vi "SLSC_Example_AsyscRTEnginer.vi"(10 "Parameters":variant, 11 "Process":refnum<class "Process.lvclass">) -> ()   [LabVIEW 2020, in "SLSC EDS Engine.lvlib"]
uses:
  SLSC EDS Engine.lvlib
  <vilib>/NI/NIVS Inline Async API/_VS Inline Async API/Process/Process.lvclass
  Types/Async Engine State Control.ctl
  Shared/Compiled.Settings
  Shared/SLSC Static Settings.ctl
  SLSC CD API/SLSC CD Engine/SLSC Dynamic Channel.ctl
  SLSC CD API/SLSC CD Engine/SLSC Datatype.ctl
  <vilib>/NI/NIVS Inline Async API/_VS Inline Async API/Process/Process.lvclass/Process.ctl
  <vilib>/NI/NIVS Inline Async API/_Data Access Engine/Access Type Classes/Read/Read.lvclass/Read.ctl
  <vilib>/NI/NIVS Inline Async API/_Data Access Engine/Access Type Classes/ReadWrite/ReadWrite.lvclass/ReadWrite.ctl
  <vilib>/NI/NIVS Inline Async API/_Data Access Engine/Access Type Classes/Write/Write.lvclass/Write.ctl
  <vilib>/NI/NIVS Inline Async API/_Data Access Engine/Data Access Engine/Methods/Read.Data.Detect.vi
  <vilib>/NI/NIVS Inline Async API/_Data Access Engine/Data Access Engine/Methods/Write.Data.vi
  <vilib>/NI/NIVS Inline Async API/_Data Access Engine/Data Access Engine/Methods/ReadWrite.Data.vi
  <vilib>/NI/NIVS Inline Async API/_VS Inline Async API/Process/Data Member Access/Read Data Access.vi
  <vilib>/NI/NIVS Inline Async API/_VS Inline Async API/Error Handling Process/SubVIs/Error.ConvertArray.vi
  <vilib>/NI/NIVS Inline Async API/_Data Access Engine/Access Type Classes/Read/Read.ProcessData.Detect.vi
  <vilib>/NI/NIVS Inline Async API/_Data Access Engine/Access Type Classes/Write/Write.ProcessData.vi
  SLSC CD API/SLSC CD Shared/SLSC Define Resource Name.vi
  <vilib>/NI/NIVS Inline Async API/_Data Access Engine/Access Type Classes/ReadWrite/ReadWrite.ProcessData.vi
  <vilib>/NI/NIVS Inline Async API/_Data Access Engine/Access Type Classes/Write/Write.Buffer.vi
  <vilib>/NI/NIVS Inline Async API/_Data Access Engine/Access Type Classes/Write/Write.Commit.vi
  Shared/Constants.vi
  <vilib>/NI/NIVS Inline Async API/_Data Access Engine/Data Access Engine/Methods/Write.Lookup.vi
  <vilib>/NI/NIVS Inline Async API/_Data Access Engine/Data Access Engine/Methods/Read.Lookup.vi
  <vilib>/NI/NIVS Inline Async API/_Data Access Engine/Data Access Engine/Methods/ReadWrite.Lookup.vi
  <vilib>/SLSC/Initialize Session with Devices.vi
  <vilib>/SLSC/Set Generic Property.vi
  <vilib>/SLSC/Set Generic Property (Bool).vi
  <vilib>/SLSC/Set Generic Property (DBL).vi
  <vilib>/SLSC/Set Generic Property (I32).vi
  <vilib>/SLSC/Set Generic Property (I64).vi
  <vilib>/SLSC/Set Generic Property (String).vi
  <vilib>/SLSC/Set Generic Property (U32).vi
  <vilib>/SLSC/Set Generic Property (U64).vi
  SLSC CD API/SLSC CD Shared/SLSC Error Suppression.vi
  <vilib>/SLSC/Commit Properties.vi
  <vilib>/SLSC/Commit Properties for Devices.vi
  <vilib>/SLSC/Execute Command.vi
  <vilib>/SLSC/Execute Device Command.vi
  <vilib>/SLSC/Execute Phys Chan Command.vi
  <vilib>/SLSC/Get Generic Property.vi
  <vilib>/SLSC/Get Generic Property (Bool).vi
  <vilib>/SLSC/Get Generic Property (DBL).vi
  <vilib>/SLSC/Get Generic Property (I32).vi
  <vilib>/SLSC/Get Generic Property (I64).vi
  <vilib>/SLSC/Get Generic Property (String).vi
  <vilib>/SLSC/Get Generic Property (U32).vi
  <vilib>/SLSC/Get Generic Property (U64).vi
  <vilib>/SLSC/Close Session.vi
  <vilib>/NI/NIVS Inline Async API/_Data Access Engine/Data Access Engine/Data Access Engine.lvclass
  <vilib>/NI VeriStand/Custom Device Tools/Custom Device Utility Library/Custom Device Utility Library.lvlib
  <vilib>/SLSC/SLSC.lvlib
  Shared/SLSC EDS Shared.lvlib
  SLSC CD API/SLSC CD Shared/SLSC CD Shared.lvlib
  SLSC CD API/SLSC CD Engine/SLSC CD Engine.lvlib
  <vilib>/NI/NIVS Inline Async API/_Data Access Engine/Access Type Classes/Write/Write.lvclass
panel:
  out "LoopRate(ms)":u32=50
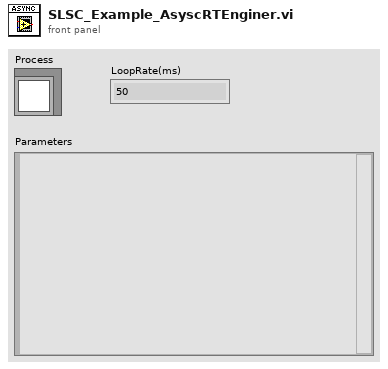
[diagram p1: front panel]
types:
  T1 = typedef "SLSC EDS Engine.lvlib/Async Engine State Control.ctl" = enum16{"Initialize", "Configure", "Run", "Reset", "Shutdown"}
  T2 = typedef "SLSC EDS Shared.lvlib/Compiled.Settings" = cluster{"Name":string, "SLSC Name or IP Address":string, "Slot #":i32, "Configuration Data":T3, "SLSC Get/Read Properties":T4[], "SLSC Set/Write Properties":T4[], "SLSC Dynamic Commands":T4[], "Support Modules":cluster{"Dev.ProductNumber":u32, "Dev.VendorNumber":u32}[]}
  T3 = typedef "SLSC EDS Shared.lvlib/SLSC Static Settings.ctl" = cluster{"Properties":cluster{"Boolean Properties":cluster{"property":refnum<k21>, "Value":bool, "SLSC Item":refnum<k21>, "reset value":bool}[], "Double Properties":cluster{"property":refnum<k21>, "Double Write":dbl, "SLSC Item":refnum<k21>, "Double Reset Value":dbl}[], "I32 Properties":cluster{"property":refnum<k21>, "Int32 Write":i32, "SLSC Item":refnum<k21>, "Int32 Reset Value":i32}[], "I64 Properties":cluster{"property":refnum<k21>, "Int64 Write":i64, "SLSC Item":refnum<k21>, "Int64 Reset Value":i64}[], "String Properties":cluster{"property":refnum<k21>, "String Write":string, "SLSC Item":refnum<k21>, "String Reset Value":string}[], "U32 Properties":cluster{"property":refnum<k21>, "UInt32 Write":u32, "SLSC Item":refnum<k21>, "UInt32 Reset Value":u32}[], "U64 Properties":cluster{"property":refnum<k21>, "UInt64 Write":u64, "SLSC Item":refnum<k21>, "UInt64 Reset Value":u64}[]}, "Commands":T4[], "Reset Commands":T4[], "Apply Values on Deployment":bool, "Apply Reset on Undeployment":bool, "Change Commands":T4[]}
  T4 = typedef "SLSC CD Shared.lvlib/SLSC Dynamic Channel.ctl" = cluster{"SLSC Item":string, "property":string, "Data Type":T5}
  T5 = typedef "SLSC CD Shared.lvlib/SLSC Datatype.ctl" = enum16{"Bool", "Double", "I32", "I64", "String", "U32", "U64"}
  T6 = typedef "Data Access Engine.lvlib/Data Access Engine.lvclass/Write.DVR.ctl" = refnum<data-value>
  T7 = typedef "Data Access Engine.lvlib/Data Access Engine.lvclass/Read.DVR.ctl" = refnum<data-value>
  T8 = typedef "Data Access Engine.lvlib/Data Access Engine.lvclass/ReadWrite.DVR.ctl" = refnum<data-value>
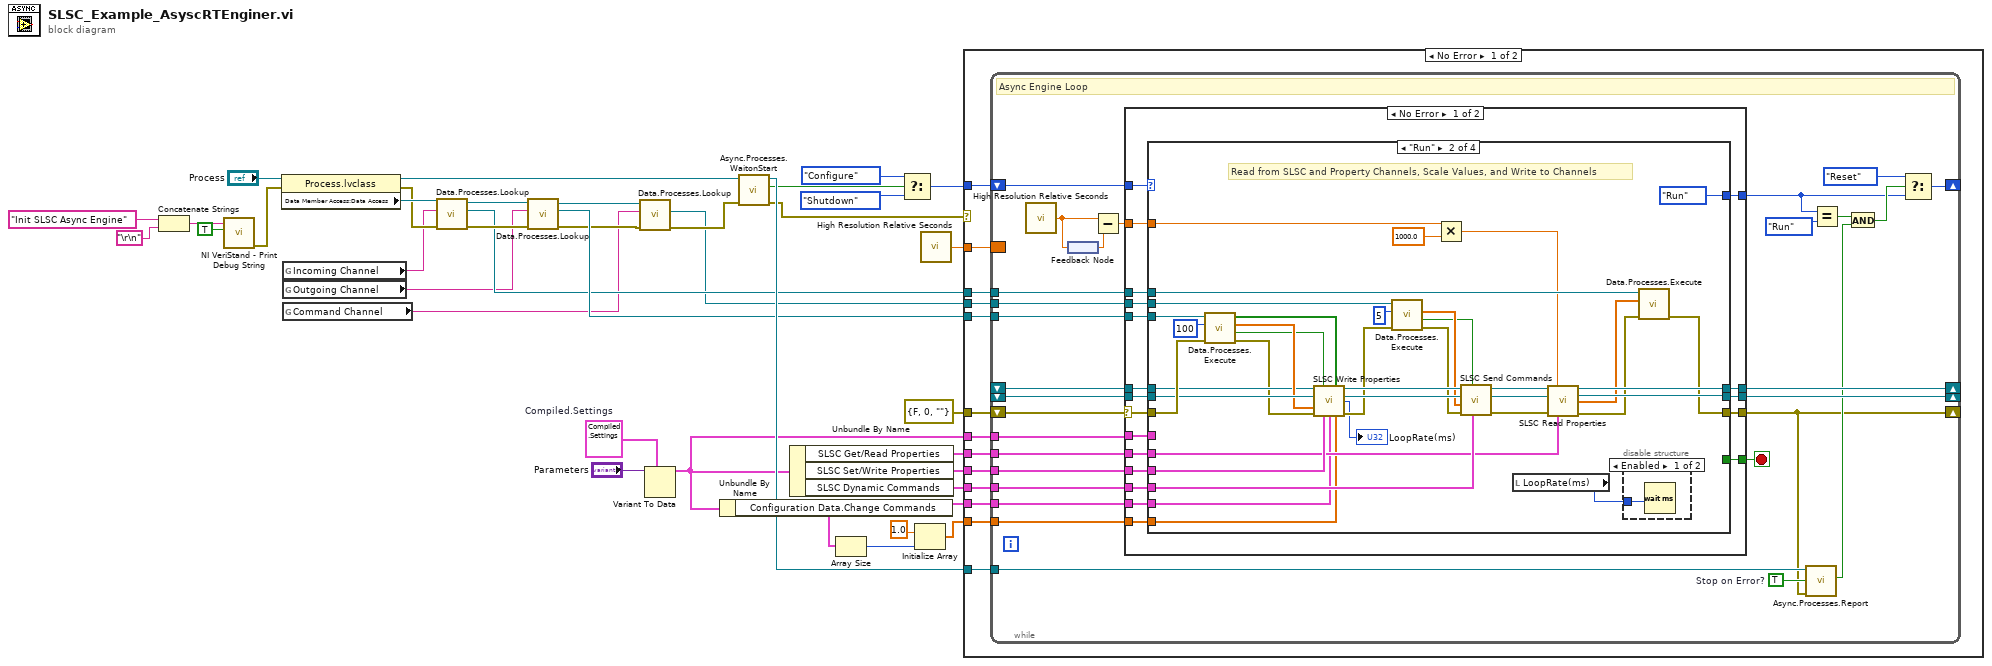
[diagram p0: block diagram]
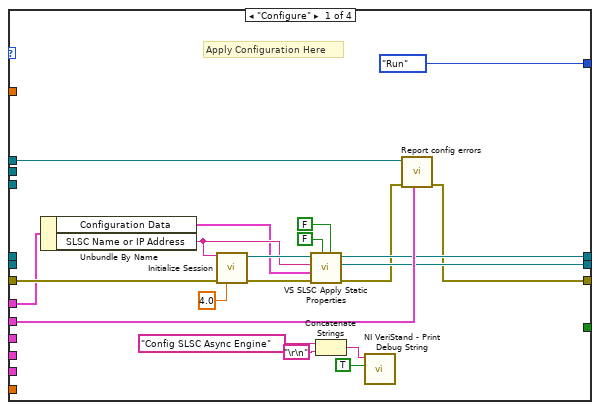
[diagram p2: hidden frame]
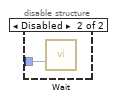
[diagram p3: hidden frame]
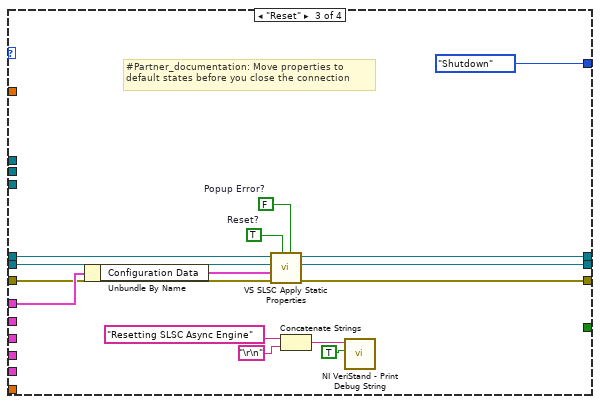
[diagram p4: hidden frame]
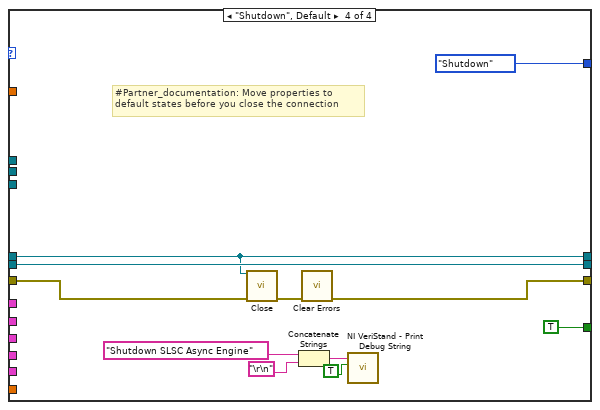
[diagram p5: hidden frame]
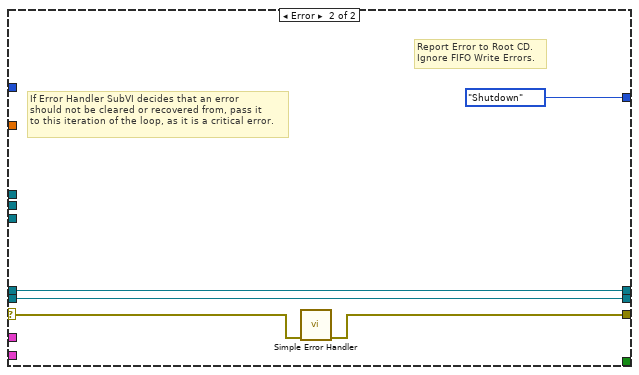
[diagram p6: hidden frame]
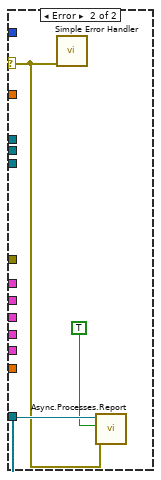
[diagram p7: hidden frame]
diagram:
  w27 = T2 {"Name"="", "SLSC Name or IP Address"="", "Slot #"=0, "Configuration Data"={"Properties"={"Boolean Properties"=[], "Double Properties"=[], "I32 Properties"=[], "I64 Properties"=[], "String Properties"=[], "U32 Properties"=[], "U64 Properties"=[]}, "Commands"=[], "Reset Commands"=[], "Apply Values on Deployment"=TRUE, "Apply Reset on Undeployment"=TRUE, "Change Commands"=[]}, "SLSC Get/Read Properties"=[], "SLSC Set/Write Properties"=[], "SLSC Dynamic Commands"=[], "Support Modules"=[]}  # Compiled.Settings
  n1 = Concatenate Strings("Init SLSC Async Engine" ("Message"), "\r\n") -> (w24:string)
  n2 = call <vilib>:"NI VeriStand - Print Debug String.vi"("Add to log file? (F)"=TRUE ("Add to log file? (T)"), "Message"=w24) -> ("error out"=w13:errorcluster)  [unwired: 9 in]
  n3 = property class="Process.lvclass"(reference="Process", error in=w13) -> (reference out=w31:refnum<class "Process.lvclass">, error out=w29:errorcluster, "Data Member Access:Data Access"=w30:refnum<class "Data Access Engine.lvclass">)
  n4 = global read "Constants.vi" "Incoming Channel"() -> (w15:string)
  n5 = global read "Constants.vi" "Outgoing Channel"() -> (w14:string)
  n6 = global read "Constants.vi" "Command Channel"() -> (w8:string)
  n7 = call-poly <vilib>:"Data.Processes.Lookup.vi"("error in (no error)"=w29, "Name"=w15, "Data Access API in"=w30) -> ("error out"=w35:errorcluster, "Ref"=w34:T6, "Data Access API out"=w33:refnum<class "Data Access Engine.lvclass">)  [unwired: 5 in, 1 out]
  n8 = call-poly <vilib>:"Data.Processes.Lookup.vi"("error in (no error)"=w35, "Name"=w14, "Data Access API in"=w33) -> ("error out"=w10:errorcluster, "Ref"=w36:T7, "Data Access API out"=w11:refnum<class "Data Access Engine.lvclass">)  [unwired: 5 in, 1 out]
  n9 = call-poly <vilib>:"Data.Processes.Lookup.vi"("error in (no error)"=w10, "Name"=w8, "Data Access API in"=w11) -> ("error out"=w9:errorcluster, "Ref"=w7:T8)  [unwired: 5 in, 2 out]
  n10 = Variant To Data(type=w27, Variant="Parameters") -> (data=w5:T2)  [unwired: 1 in, 1 out]
  n11 = Unbundle By Name(w5) -> ("Configuration Data.Change Commands"=w4:T4[])
  n12 = call <vilib>:"Async.Processes.WaitonStart.vi"("error in (no error)"=w9, "Process"=w31) -> ("error out"=w37:errorcluster, "Execute"=w21:bool, "Process out"=w38:refnum<class "Process.lvclass">)  [unwired: 7 in]
  n13 = Unbundle By Name(w5) -> ("SLSC Get/Read Properties"=w17:T4[], "SLSC Set/Write Properties"=w16:T4[], "SLSC Dynamic Commands"=w12:T4[])
  n14 = Array Size(array=w4) -> (size(s)=w2:i32)
  n15 = Select(t=Async_Engine_State_Control."Configure", s=w21, f=Async_Engine_State_Control."Shutdown") -> (s? t:f=w18:T1)
  n16 = Initialize Array(1.0 ("element"), w2) -> (w1:dbl[])
  n17 = call <vilib>:"High Resolution Relative Seconds.vi"() -> ("relative seconds"=w6:dbl)
  n18 = case shown="No Error" w37 {
    selector: w37 -> [_ w191]
    tunnel: w38 -> [w51 w192]
    tunnel: w34 -> [w50 _]
    tunnel: w36 -> [w49 _]
    tunnel: w5 -> [w44 _]
    tunnel: errorcluster {"status"=FALSE, "code"=0, "source"=""} ("error IO") -> [w41 _]
    tunnel: w18 -> [w48 _]
    tunnel: w17 -> [w47 _]
    tunnel: w16 -> [w46 _]
    tunnel: w6 -> [w45 _]
    tunnel: w12 -> [w43 _]
    tunnel: w7 -> [w42 _]
    tunnel: w4 -> [w40 _]
    tunnel: w1 -> [w39 _]
    frame No Error {
      n19 = while {
        shift-right: [w55] -> _
        shift-left: w41 -> [w80]
        shift-right: [w63] -> _
        shift-left: w48 -> [w79]
        shift-right: [w77] -> _
        shift-left: _ -> [w76]
        tunnel: w49 -> [w75]
        tunnel: w50 -> [w74]
        tunnel: w51 -> [w73]
        tunnel: w47 -> [w72]
        tunnel: w46 -> [w71]
        shift-right: [w70] -> _
        shift-left: _ -> [w69]
        border: w45 -> [_]
        tunnel: w43 -> [w62]
        tunnel: w42 -> [w61]
        tunnel: w44 -> [w78]
        tunnel: w40 -> [w53]
        tunnel: w39 -> [w52]
        stop <- w65 stop-if-true
        w68 = TRUE  # Stop on Error?
        # "Async Engine Loop"
        n20 = call <vilib>:"High Resolution Relative Seconds.vi"() -> ("relative seconds"=w54:dbl)
        n21 = feedback-in #1(w54) -> ()
        n22 = feedback #1() -> (w67:dbl)
        n23 = Subtract(x=w54, y=w67) -> (x-y=w66:dbl)
        n24 = case shown="No Error" w80 {
          selector: w80 -> [w98 w186]
          tunnel: [w92 w185] -> w55
          tunnel: w79 -> [w99 _]
          tunnel: [w93 Async_Engine_State_Control."Shutdown"] -> w59
          tunnel: [w97 _] -> w65
          tunnel: w78 -> [w96 _]
          tunnel: [w95 w189] -> w77
          tunnel: w76 -> [w94 w189]
          tunnel: w75 -> [w91 _]
          tunnel: w74 -> [w90 _]
          tunnel: w72 -> [w89 _]
          tunnel: w71 -> [w88 _]
          tunnel: [w87 w187] -> w70
          tunnel: w69 -> [w86 w187]
          tunnel: w66 -> [w85 _]
          tunnel: w62 -> [w84 _]
          tunnel: w61 -> [w83 _]
          tunnel: w53 -> [w82 _]
          tunnel: w52 -> [w81 _]
          frame No Error {
            n25 = case shown="\"Run\"" w99 {
              tunnel: w98 -> [w119 w154 w167 w175]
              tunnel: [w101 w127 w166 w177] -> w92
              tunnel: [Async_Engine_State_Control."Run" Async_Engine_State_Control."Run" Async_Engine_State_Control."Shutdown" Async_Engine_State_Control."Shutdown"] -> w93
              tunnel: [_ _ _ TRUE] -> w97
              tunnel: w96 -> [w113 _ w168 _]
              tunnel: [w110 w147 w160 w176] -> w95
              tunnel: w94 -> [_ w152 w162 w176]
              tunnel: w91 -> [_ w155 _ _]
              tunnel: w90 -> [w112 w131 _ _]
              tunnel: w89 -> [w111 w130 _ _]
              tunnel: w88 -> [_ w150 _ _]
              tunnel: [w109 w148 w161 w174] -> w87
              tunnel: w86 -> [_ w149 w163 w174]
              tunnel: w85 -> [_ w128 _ _]
              tunnel: w84 -> [_ w137 _ _]
              tunnel: w83 -> [_ w129 _ _]
              tunnel: w82 -> [_ w121 _ _]
              tunnel: w81 -> [_ w120 _ _]
              frame "Configure" {
                # "Apply Configuration Here"
                n26 = Unbundle By Name(w113) -> ("Configuration Data"=w100:T3, "SLSC Name or IP Address"=w104:string)
                n27 = call-poly <vilib>:"Initialize Session.vi"("devices"=w104, "error in (no error)"=w119, "connect timeout (60 sec)"=4.0 ("connect timeout (10 sec)")) -> ("session out"=w106:refnum<k21>, "error out"=w105:errorcluster)  [unwired: 11 in]
                n28 = call "VS SLSC Apply Static Properties.vi"("Popup Error?"=FALSE, "Reset?"=FALSE, "error in (no error)"=w105, "Configuration Data"=w100, "SLSC Module Name in"=w104, "Refnum in"=w106) -> ("error out"=w102:errorcluster, "SLSC Module Name out"=w110:refnum<k21>, "Refnum out"=w109:refnum<k21>)  [unwired: 3 in]
                n29 = Concatenate Strings("Config SLSC Async Engine" ("Message"), "\r\n") -> (w115:string)
                n30 = call <vilib>:"NI VeriStand - Print Debug String.vi"("Add to log file? (F)"=TRUE ("Add to log file? (T)"), "Message"=w115) -> ()  [unwired: 9 in, 1 out]
                n31 = call "Report config errors.vi"("SLSC Dynamic Inputs"=w111, "error in (no error)"=w102, "Data Value Reference in"=w112) -> ("error out"=w101:errorcluster)  [unwired: 8 in]
              }
              frame "Run" {
                # "Read from SLSC and Property Channels, Scale Values, and Write to Channels"
                n32 = call-poly <vilib>:"Data.Processes.Execute.vi"("error in (no error)"=w154, "timeout ms"=100, "Ref"=w155) -> ("error out"=w136:errorcluster, "Timeout?"=w133:bool, "Values"=w151:dbl[], "Detect?"=w122:bool[])  [unwired: 5 in]
                n33 = call "SLSC Write Properties.vi"("session in"=w149, "Stop Updating?"=w133, "Detect?"=w122, "SLSC Module Name"=w152, "Values"=w151, "error in"=w136, "SLSC Dynamic Outputs"=w150, "Change Commands"=w121, "Command Values"=w120) -> ("session out"=w143:refnum<k21>, "SLSC Module Name"=w142:refnum<k21>, "LoopRate(ms)"=→"LoopRate(ms)":u32, "error out"=w135:errorcluster)  [unwired: 3 in]
                n34 = call-poly <vilib>:"Data.Processes.Execute.vi"("error in (no error)"=w135, "timeout ms"=5, "Ref"=w129) -> ("error out"=w134:errorcluster, "Timeout?"=w132:bool, "Data"=w139:dbl[])  [unwired: 5 in, 1 out]
                n35 = Multiply(x=w128, y=1000.0) -> (x*y=w126:dbl)
                n36 = call "SLSC Send Commands.vi"("SLSC Dynamic Commands"=w137, "Timeout?"=w132, "error in"=w134, "Values"=w139, "SLSC Module Name"=w142, "session in"=w143) -> ("error out"=w138:errorcluster, "SLSC Module Name"=w140:refnum<k21>, "session out"=w141:refnum<k21>)  [unwired: 3 in]
                n37 = local read "LoopRate(ms)"() -> (w123:u32)
                n38 = call "SLSC Read Properties.vi"("session in"=w141, "LoopDuration(ms)"=w126, "SLSC Module Name"=w140, "error in"=w138, "SLSC Dynamic Inputs"=w130) -> ("session out"=w148:refnum<k21>, "SLSC Module Name"=w147:refnum<k21>, "Values"=w145:dbl[], "error out"=w146:errorcluster)  [unwired: 7 in]
                n39 = disable-structure shown="Enabled" {
                  disable-tunnel: w123 -> [w157 w158]
                  frame Enabled {
                    n40 = Wait (ms)(milliseconds to wait=w157) -> ()  [unwired: 1 out]
                  }
                  frame Disabled {
                    n41 = call "Wait"("Count(mSec)"=w158) -> ()  [unwired: 1 out]
                  }
                }
                n42 = call-poly <vilib>:"Data.Processes.Execute.vi"("error in (no error)"=w146, "Values"=w145, "Ref"=w131) -> ("error out"=w127:errorcluster)  [unwired: 8 in]
              }
              frame "Reset" {
                w159 = FALSE  # Popup Error?
                w164 = TRUE  # Reset?
                # "#Partner_documentation: Move properties to \ndefault states before you close the connection"
                n43 = Unbundle By Name(w168) -> ("Configuration Data"=w165:T3)
                n44 = call "VS SLSC Apply Static Properties.vi"("Popup Error?"=w159, "Reset?"=w164, "error in (no error)"=w167, "Configuration Data"=w165, "SLSC Module Name in"=w162, "Refnum in"=w163) -> ("error out"=w166:errorcluster, "SLSC Module Name out"=w160:refnum<k21>, "Refnum out"=w161:refnum<k21>)  [unwired: 3 in]
                n45 = Concatenate Strings("Resetting SLSC Async Engine" ("Message"), "\r\n") -> (w170:string)
                n46 = call <vilib>:"NI VeriStand - Print Debug String.vi"("Add to log file? (F)"=TRUE ("Add to log file? (T)"), "Message"=w170) -> ()  [unwired: 9 in, 1 out]
              }
              frame "Shutdown", Default {
                # "#Partner_documentation: Move properties to \ndefault states before you close the connection"
                n47 = call-poly <vilib>:"Close.vi"("session in"=w174, "error in (no error)"=w175) -> ("error out"=w178:errorcluster)  [unwired: 13 in]
                n48 = Concatenate Strings("Shutdown SLSC Async Engine" ("Message"), "\r\n") -> (w180:string)
                n49 = call <vilib>:"Clear Errors.vi"("error in (no error)"=w178) -> ("error out"=w177:errorcluster)  [unwired: 5 in, 1 out]
                n50 = call <vilib>:"NI VeriStand - Print Debug String.vi"("Add to log file? (F)"=TRUE ("Add to log file? (T)"), "Message"=w180) -> ()  [unwired: 9 in, 1 out]
              }
            }
          }
          frame Error {
            # "If Error Handler SubVI decides that an error\nshould not be cleared or recovered from, pass it\nto this iteration of the loop, as it is a critical error."
            # "Report Error to Root CD.\nIgnore FIFO Write Errors."
            n51 = call <vilib>:"Simple Error Handler.vi"("error in (no error)"=w186) -> ("error out"=w185:errorcluster)  [unwired: 4 in, 4 out]
          }
        }
        n52 = call <vilib>:"Async.Processes.Report.vi"("Error"=w55, "Stop Async on Error?"=w68, "Process in"=w73) -> ("Stop"=w64:bool)  [unwired: 7 in, 1 out]
        n53 = Equal?(x=w59, y=Async_Engine_State_Control."Run") -> (x = y?=w58:bool)
        n54 = And(x=w58, y=w64) -> (x .and. y?=w60:bool)
        n55 = Select(t=Async_Engine_State_Control."Reset", s=w60, f=w59) -> (s? t:f=w63:T1)
      }
    }
    frame Error {
      n56 = call <vilib>:"Simple Error Handler.vi"("error in (no error)"=w191) -> ()  [unwired: 4 in, 5 out]
      n57 = call <vilib>:"Async.Processes.Report.vi"("Error"=w191, "Stop Async on Error?"=TRUE ("Stop on Error?"), "Process in"=w192) -> ()  [unwired: 7 in, 2 out]
    }
  }
